vi "RH_Relays_Close.vi"(8 "error in":errorcluster, 11 "Relays Session In":refnum<k15>) -> (0 "error out":errorcluster)   [LabVIEW 2023, in "ResourceHandling.lvlib"]
doc: "Disconnect and Close the relay driver session"
uses:
  ResourceHandling.lvlib
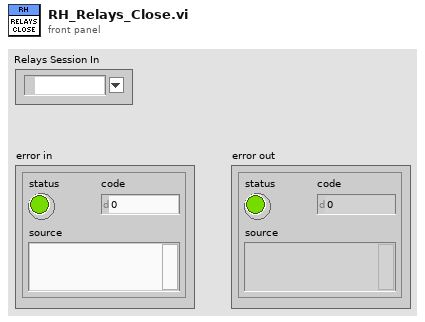
[diagram p1: front panel]
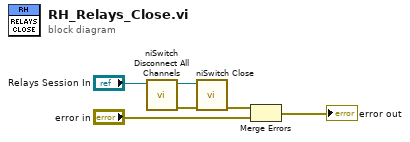
[diagram p0: block diagram]
diagram:
  n1 = call <instrlib>:"niSwitch Disconnect All Channels.vi"("instrument handle"="Relays Session In") -> ("error out"=w5:errorcluster, "instrument handle out"=w4:refnum<k15>)  [unwired: 9 in]
  n2 = call <instrlib>:"niSwitch Close.vi"("error in (no error)"=w5, "instrument handle"=w4) -> ("error out"=w6:errorcluster)  [unwired: 9 in]
  n3 = Merge Errors(w6, "error in") -> (→"error out":errorcluster)
